vi "Set DDG Times.vi"(9 "t2":dbl, 10 "t1":dbl, 11 "t0":dbl) -> (3 "function return":u32)   [LabVIEW 2018, in "Copy of Andor SDK.lvlib"]
doc: "EXPNETTYPE unsigned int WINAPI SetDDGTimes(double t0, double t1, double t2);"
uses:
  Copy of Andor SDK.lvlib
  <userlib>/Andor SDK/ATMCD32D.dll
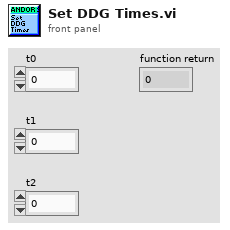
[diagram p1: front panel]
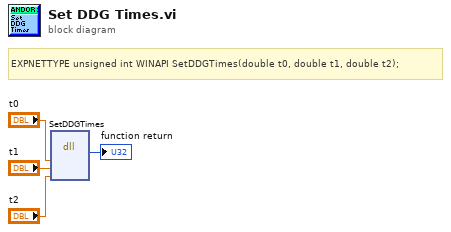
[diagram p0: block diagram]
diagram:
  # "EXPNETTYPE unsigned int WINAPI SetDDGTimes(double t0, double t1, double t2);"
  n1 = dll-call lib="C:/Program Files (x86)/National Instruments/LabVIEW 2018/user.lib/Andor SDK/ATMCD32D.*" fn="SetDDGTimes"("t0"="t0", "t1"="t1", "t2"="t2") -> (→"function return":u32)  [unwired: 6 in, 2 out]
